vi "Add RTV.vi"(0 "RT Variables in":refnum<class "RT Variables.lvclass">, 5 "RTV name":string, 7 "Data":variant, 9 "Scope":i64, 11 "error in (no error)":errorcluster) -> (4 "RT Variables out":refnum<class "RT Variables.lvclass">, 15 "error out":errorcluster)   [LabVIEW 2016, in "RT Variables.lvclass"]
uses:
  RT Variables.lvclass
  RT Variables.lvclass/RT Variables.ctl
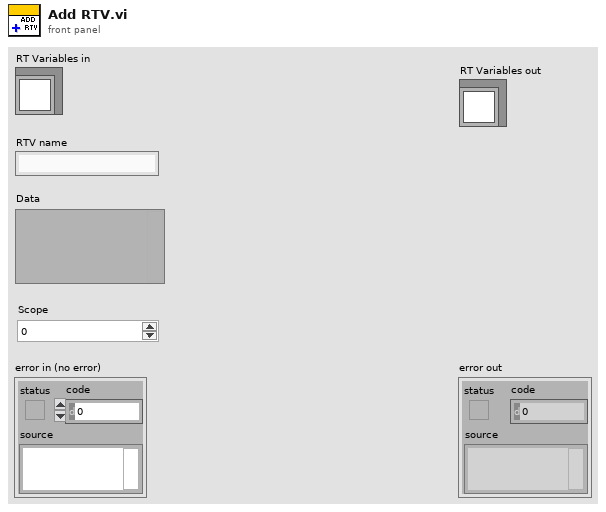
[diagram p1: front panel]
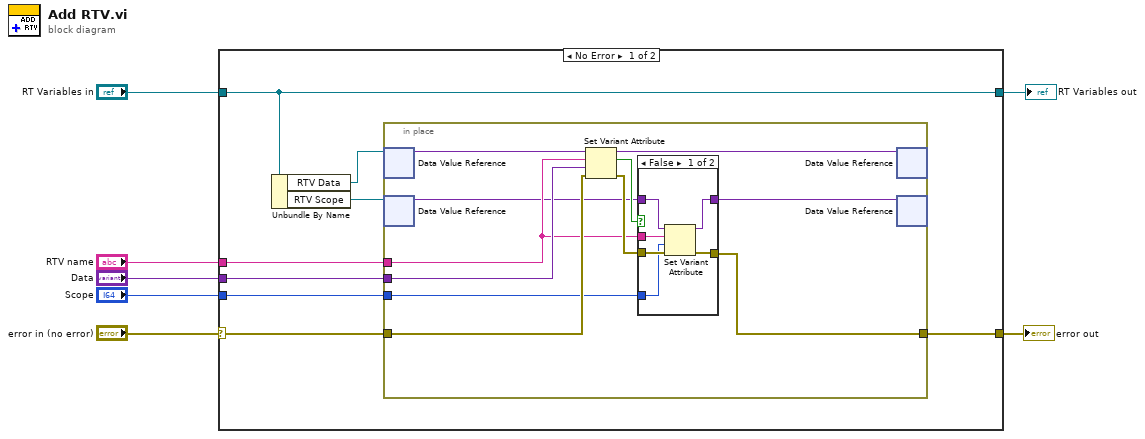
[diagram p0: block diagram]
diagram:
  n1 = case shown="No Error" "error in (no error)" {
    selector: "error in (no error)" -> [w15 w36]
    tunnel: [w13 w36] -> w6
    tunnel: "RTV name" -> [w12 _]
    tunnel: "Data" -> [w14 _]
    tunnel: "Scope" -> [w11 _]
    tunnel: "RT Variables in" -> [w8 w35]
    tunnel: [w8 w35] -> w1
    frame No Error {
      n2 = Unbundle By Name(w8) -> ("RTV Data"=w10:refnum<data-value>, "RTV Scope"=w9:refnum<data-value>)
      n3 = in-place {
        in-place-border: w15 -> [w26]
        in-place-border: w14 -> [w25]
        in-place-border: [w23] -> w13
        in-place-border: w12 -> [w22]
        in-place-border: w11 -> [w21]
        n4 = in-place-dvr #1(w10) -> (w17:variant)  [unwired: 1 out]
        n5 = in-place-dvr #2(w9) -> (w19:variant)  [unwired: 1 out]
        n6 = Set Variant Attribute(Variant=w17, name=w22, value=w25, error in=w26) -> (Variant out=w16:variant, replaced=w20:bool, error out=w24:errorcluster)
        n7 = case shown="False" w20 {
          tunnel: w19 -> [w32 w33]
          tunnel: [w31 w33] -> w18
          tunnel: w24 -> [w30 w34]
          tunnel: [w29 w34] -> w23
          tunnel: w22 -> [w28 _]
          tunnel: w21 -> [w27 _]
          frame False {
            n8 = Set Variant Attribute(Variant=w32, name=w28, value=w27, error in=w30) -> (Variant out=w31:variant, error out=w29:errorcluster)  [unwired: 1 out]
          }
          frame True {
          }
        }
        n9 = in-place-dvr #1(w16) -> ()  [unwired: 2 out]
        n10 = in-place-dvr #2(w18) -> ()  [unwired: 2 out]
      }
    }
    frame Error {
    }
  }
  "error out" <- w6
  "RT Variables out" <- w1
